vi "Set Vecto Info.vi"(8 "error in (no error)":errorcluster, 11 "System Config Module in":refnum<class "System Config Module.lvclass">) -> (0 "error out":errorcluster, 3 "System Config Module out":refnum<class "System Config Module.lvclass">)   [LabVIEW 2020, in "Volatus.lvlib" / "System Config Module.lvclass"]
uses:
  System Config Module.lvclass
  System Config Module.lvclass/System Config Module.ctl
  lv-builder/Builder Core/Builder Core.lvlib
  Module/Module.lvclass
  VolatusAPI/VolatusAPI.lvclass
  C:/dev/lv20CE/relink/lv-volatus/Volatus/Module/Module.lvclass
  C:/dev/lv20CE/relink/lv-volatus/Volatus/System Config Server/System Config Module.lvclass
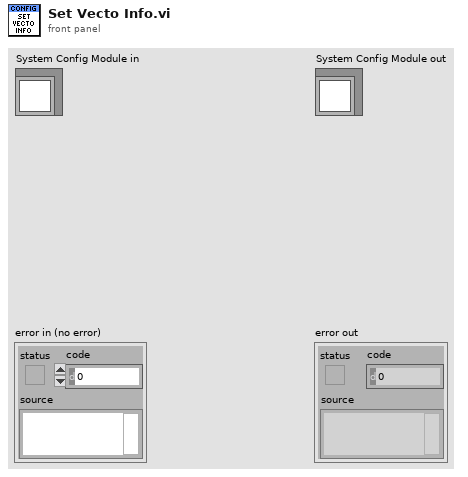
[diagram p1: front panel]
types:
  T1 = typedef "Builder Core.lvlib/Version.ctl" = cluster{"Major":u16, "Minor":u16, "Fix":u16, "Build":u16}
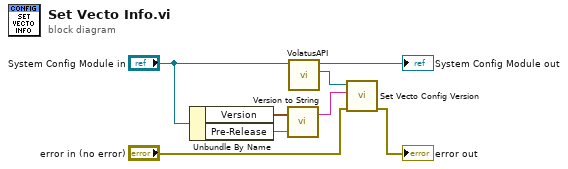
[diagram p0: block diagram]
diagram:
  n1 = Unbundle By Name("System Config Module in") -> ("Version"=w7:T1, "Pre-Release"=w6:string)
  n2 = call "Version to String.vi"("Version"=w7, "Pre-Release (None)"=w6) -> ("Version String"=w3:string)  [unwired: 5 in]
  n3 = call "VolatusAPI.vi"("Module in"="System Config Module in") -> ("VolatusAPI"=w4:refnum<class "VolatusAPI.lvclass">, "Module out"=→"System Config Module out":refnum<class "System Config Module.lvclass">)  [unwired: 9 in]
  n4 = call "Set Vecto Config Version.vi"("error in (no error)"="error in (no error)", "Cfg Version"=w3, "VolatusAPI in"=w4) -> ("error out"=→"error out":errorcluster)  [unwired: 7 in, 1 out]
